vi "chamber_indicator.vi"(9 "bullet amount":u32, 10 "empty round":u32, 11 "live round":u32) -> (3 "picture":u32[](array[ring]))   [LabVIEW 2025]
panel:
  out "chamber":u32[](array[numeric])
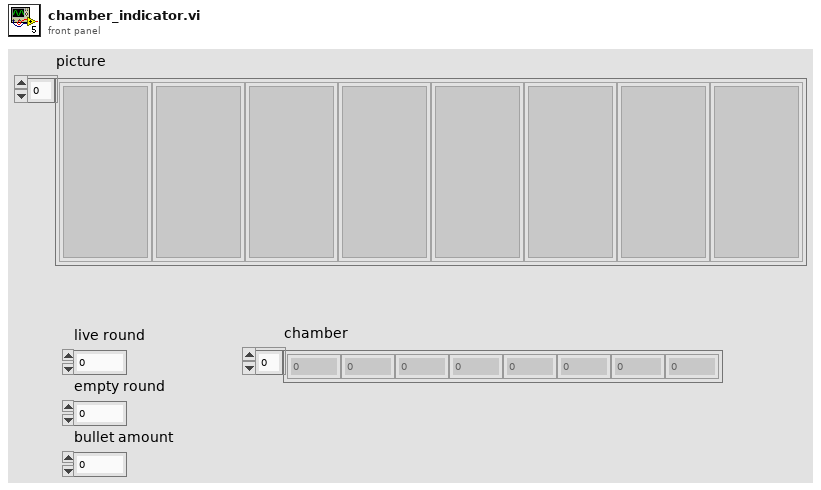
[diagram p1: front panel]
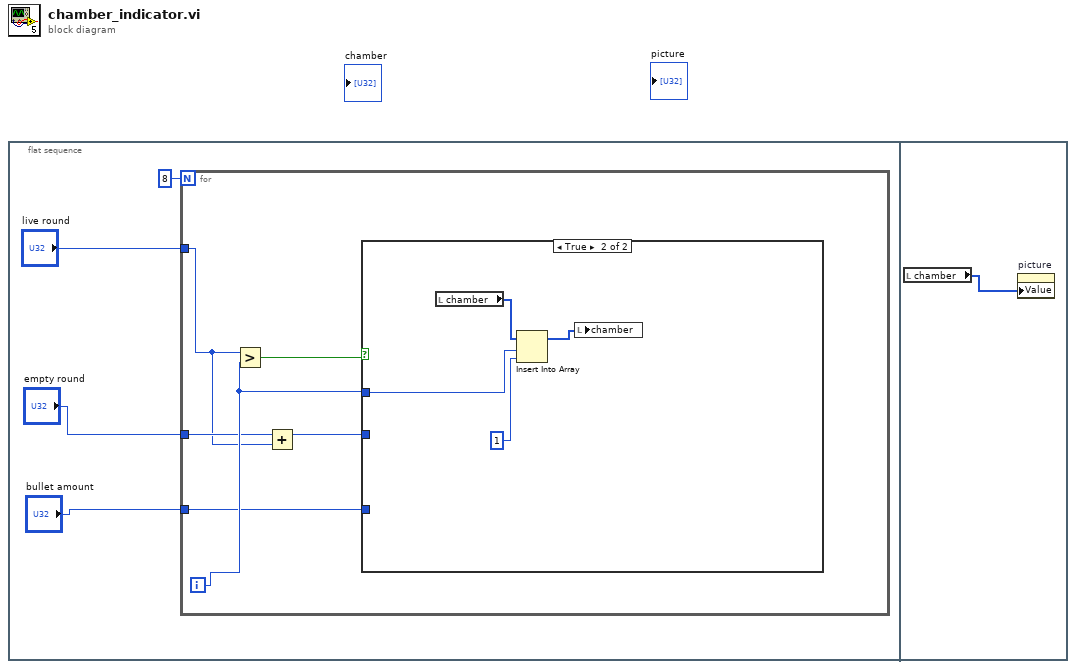
[diagram p0: block diagram]
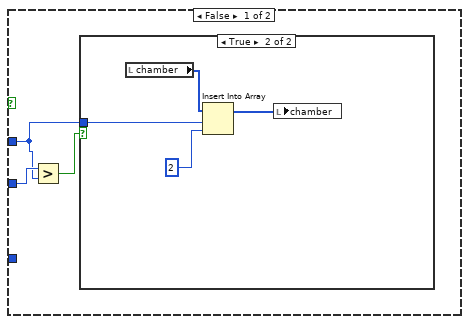
[diagram p2: hidden frame]
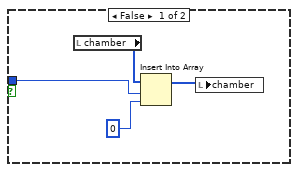
[diagram p3: hidden frame]
diagram:
  n1 = flat-sequence {
    frame #0 {
      n2 = for {
        N: 8 -> [_]
        tunnel: "live round" -> [w6]
        tunnel: "empty round" -> [w8]
        tunnel: "bullet amount" -> [w5]
        i -> [w9]
        n3 = Greater?(x=w6, y=w9) -> (0:w10:bool)
        n4 = Add(x=w8, y=w6) -> (x+y=w7:u32)
        n5 = case shown="True" w10 {
          tunnel: w9 -> [w11 w25]
          tunnel: w7 -> [w12 _]
          tunnel: w5 -> [_ _]
          frame False {
            n6 = Greater?(x=w12, y=w11) -> (0:w13:bool)
            n7 = case shown="True" w13 {
              tunnel: w11 -> [w17 w21]
              frame False {
                n8 = local read "chamber"() -> (w14:u32[])
                n9 = Insert Into Array(array=w14, index=w17, new element=u32 0 ("new element/subarray")) -> (w15:u32[])
                n10 = local write "chamber"(w15) -> ()
              }
              frame True {
                n11 = local read "chamber"() -> (w18:u32[])
                n12 = Insert Into Array(array=w18, index=w21, new element=u32 2 ("new element/subarray")) -> (w19:u32[])
                n13 = local write "chamber"(w19) -> ()
              }
            }
          }
          frame True {
            n14 = local read "chamber"() -> (w22:u32[])
            n15 = Insert Into Array(array=w22, index=w25, new element=u32 1 ("new element/subarray")) -> (w23:u32[])
            n16 = local write "chamber"(w23) -> ()
          }
        }
      }
    }
    frame #1 {
      n17 = local read "chamber"() -> (w26:u32[])
      n18 = property on="picture" class="Arr (strict)"("Value"=w26) -> ()  [unwired: 2 in, 2 out]
    }
  }
